vi "P9-P14TMonitor.vi"() -> ()   [LabVIEW 2019]
uses:
  Utility/Monitor Communication/PPMS/P9P14-TCluster.ctl
  Instrument_Setup.vi
  Global/Global Variables/Data_Display_global.vi
panel:
  in  "stop":bool
  in  "InstrumentType":i32(ring) items=["PPMS", "VersaLab", "DynaCool", "SVSM", "OptiCool"]
  in  "Remote":bool
  out "P9-P14 T-Cluster":T1 {"Temperature\nStatus" items=["TemperatureUnknown"=0, "Stable"=1, "Tracking"=2, "Near"=5, "Chasing"=6, "Filling"=7, "Standby"=10, "Disabled"=13, "ImpedanceNotFunction"=14, "TempFailure"=15]; "Approach" items=["Fast Settle", "No O'Shoot"]}
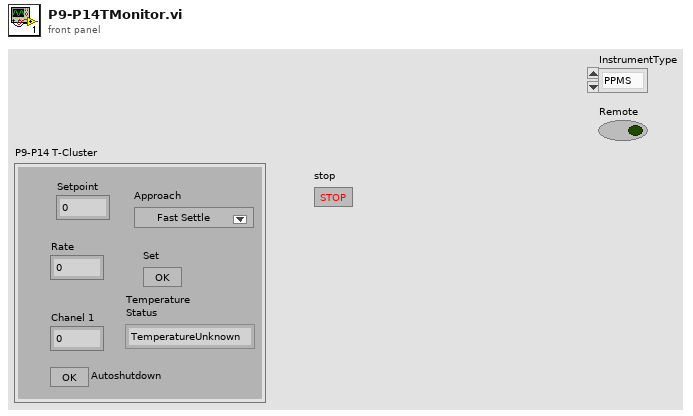
[diagram p1: front panel]
types:
  T1 = typedef "P9P14-TCluster.ctl" = cluster{"Setpoint":dbl, "Rate":dbl, "Chanel 1":dbl, "Approach":u16, "Set":bool, "Temperature\nStatus":i32, "Autoshutdown":bool}
  T2 = typedef "P9P14-TCluster-Control.ctl" = cluster{"Setpoint":dbl, "Rate":dbl, "Approach":u16, "Set":bool, "Autoshutdown":bool}
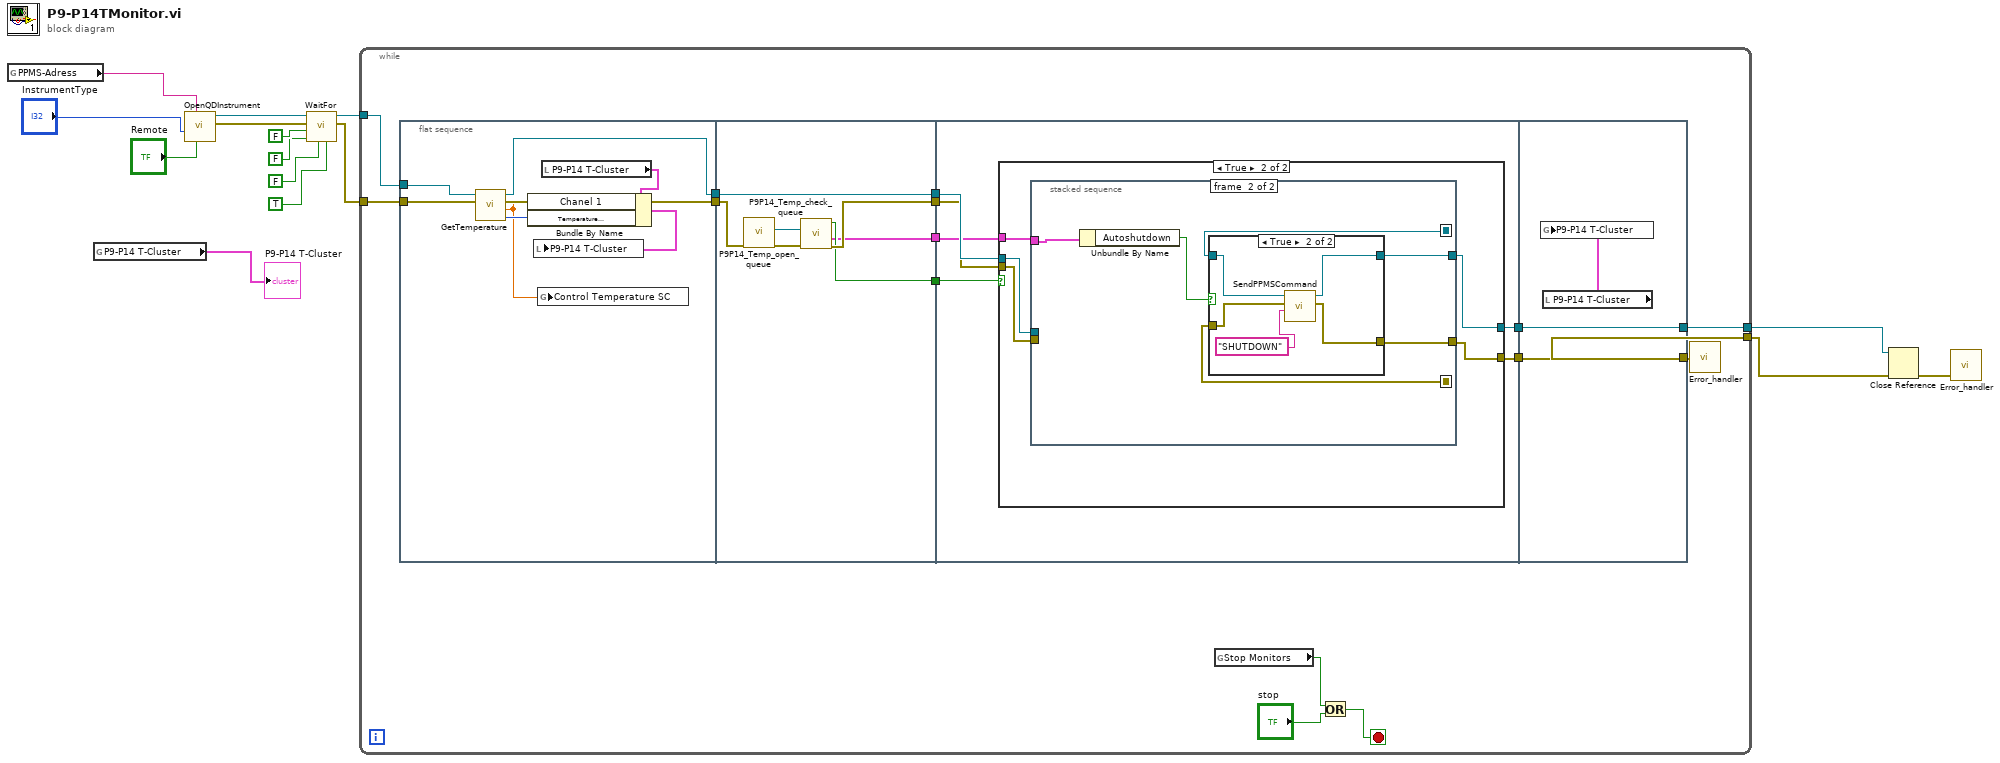
[diagram p0: block diagram]
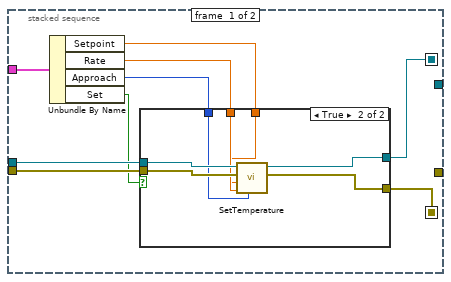
[diagram p3: hidden frame]
diagram:
  n1 = global read "Instrument_Setup.vi" "PPMS-Adress"() -> (w7:string)
  n2 = global read "Data_Display_global.vi" "P9-P14 T-Cluster"() -> (→"P9-P14 T-Cluster":T1)
  n3 = call "OpenQDInstrument.vi"("Remote"="Remote", "IP Address"=w7, "InstrumentType"="InstrumentType") -> ("error out"=w8:errorcluster, "Instrument Ref"=w9:refnum<k24>)  [unwired: 5 in]
  n4 = call "WaitFor.vi"("Wait For Chamber"=TRUE ("WaitForChamber"), "Wait For Position"=FALSE ("WaitForPosition"), "Wait For Field"=FALSE ("WaitForField"), "Wait For Temperature"=FALSE ("WaitForTemperature"), "error in (no error)"=w8, "Instrument Ref In"=w9) -> ("error out"=w6:errorcluster, "Instrument Ref Out"=w5:refnum<k24>)  [unwired: 4 in]
  n5 = while {
    tunnel: w6 -> [w27]
    tunnel: w5 -> [w26]
    tunnel: [w19] -> w2
    tunnel: [w18] -> w4
    stop <- w30 stop-if-true
    n6 = flat-sequence {
      tunnel: w27 -> [w38]
      tunnel: w26 -> [w37]
      tunnel: [w33] -> w24
      tunnel: [w32] -> w22
      tunnel: [w45] -> w25
      tunnel: w24 -> [w45]
      tunnel: [w42] -> w23
      tunnel: w22 -> [w44]
      tunnel: [w40] -> w21
      tunnel: [w39] -> w20
      tunnel: w25 -> [w51]
      tunnel: w23 -> [w50]
      tunnel: w21 -> [w49]
      tunnel: w20 -> [w48]
      tunnel: [w47] -> w17
      tunnel: [w46] -> w16
      tunnel: [w91] -> w18
      tunnel: [w92] -> w19
      tunnel: w17 -> [w92]
      tunnel: w16 -> [w91]
      frame #0 {
        n7 = call "GetTemperature.vi"("error in (no error)"=w38, "Instrument Ref In"=w37) -> ("Temperature\nStatus"=w34:i32, "Temperature"=w31:dbl, "error out"=w32:errorcluster, "Instrument Ref Out"=w33:refnum<k24>)  [unwired: 3 in, 1 out]
        n8 = global write "Data_Display_global.vi" "Control Temperature SC"(w31) -> ()
        n9 = local read "P9-P14 T-Cluster"() -> (w36:T1)
        n10 = Bundle By Name(cluster=w36, "Chanel 1"=w31, "Temperature\nStatus"=w34) -> (w35:T1)
        n11 = local write "P9-P14 T-Cluster"(w35) -> ()
      }
      frame #1 {
        n12 = call "P9P14_Temp_open_queue.vi"("error in (no error)"=w44) -> ("error out"=w43:errorcluster, "queue out"=w41:refnum<queue>)  [unwired: 9 in]
        n13 = call "P9P14_Temp_check_queue.vi"("error in (no error)"=w43, "Queue"=w41) -> ("error out"=w42:errorcluster, "P9-P14 T-Cluster -Control"=w39:T2, "New Entries?"=w40:bool)  [unwired: 7 in]
      }
      frame #2 {
        n14 = case shown="True" w49 {
          tunnel: w51 -> [w53 w58]
          tunnel: w50 -> [w52 w57]
          tunnel: w48 -> [_ w56]
          tunnel: [w52 w54] -> w47
          tunnel: [w53 w55] -> w46
          frame False {
          }
          frame True {
            n15 = stacked-sequence {
              seq-local: [w60 _] -> [_ w80]
              seq-local: [w59 _] -> [_ w81]
              tunnel: w58 -> [w67 _]
              tunnel: w57 -> [w66 _]
              tunnel: w56 -> [w65 w82]
              tunnel: [_ w78] -> w55
              tunnel: [_ w77] -> w54
              frame #0 {
                n16 = Unbundle By Name(w65) -> ("Setpoint"=w62:dbl, "Rate"=w63:dbl, "Approach"=w61:u16, "Set"=w64:bool)
                n17 = case shown="True" w64 {
                  tunnel: w67 -> [w69 w76]
                  tunnel: w66 -> [w68 w75]
                  tunnel: w63 -> [_ w74]
                  tunnel: w62 -> [_ w73]
                  tunnel: w61 -> [_ w72]
                  tunnel: [w68 w71] -> w60
                  tunnel: [w69 w70] -> w59
                  frame False {
                  }
                  frame True {
                    n18 = call "SetTemperature.vi"("Approach"=w72, "Rate"=w74, "Temperature"=w73, "error in (no error)"=w75, "Instrument Ref In"=w76) -> ("error out"=w71:errorcluster, "Instrument Ref Out"=w70:refnum<k24>)  [unwired: 2 in, 1 out]
                  }
                }
              }
              frame #1 {
                n19 = Unbundle By Name(w82) -> ("Autoshutdown"=w79:bool)
                n20 = case shown="True" w79 {
                  tunnel: w81 -> [w84 w89]
                  tunnel: w80 -> [w83 w86]
                  tunnel: [w84 w88] -> w78
                  tunnel: [w83 w87] -> w77
                  frame False {
                  }
                  frame True {
                    n21 = call "SendPPMSCommand.vi"("PpmsCommand"="SHUTDOWN", "error in (no error)"=w86, "Instrument Ref In"=w89) -> ("error out"=w87:errorcluster, "Instrument Ref Out"=w88:refnum<k24>)  [unwired: 4 in, 3 out]
                  }
                }
              }
            }
          }
        }
      }
      frame #3 {
        n22 = local read "P9-P14 T-Cluster"() -> (w90:T1)
        n23 = global write "Data_Display_global.vi" "P9-P14 T-Cluster"(w90) -> ()
      }
    }
    n24 = global read "Data_Display_global.vi" "Stop Monitors"() -> (w29:bool)
    n25 = Or(x=w29, y="stop") -> (x .or. y?=w30:bool)
    n26 = call "Error_handler.vi"("error constant"=w19) -> ()
  }
  n27 = Close Reference(reference=w4, error in (no error)=w2) -> (error out=w3:errorcluster)
  n28 = call "Error_handler.vi"("error constant"=w3) -> ()
